vi "Update ROI times.vi"(11 "ROI setup in":T1[](array[typedef]) {"ROI group ID" format="%#_6f"; "Laser Power (%)" format="%#_6f"; "Zoom" format="%#_6f"; "Frame Size" format="%#_6f"; "Number of lines" format="%#_6f"; "Composite ID" format="%#_6f"; "Angle (deg)" format="%#_6f"; "ROI Time (ns)" format="%#_6f"; "ROI ID" format="%#_6f"; "Pixels in ROI" format="%#_6f"; "ROI index" format="%#_6f"; "Z stop" format="%#_6f"; "Y stop" format="%#_6f"; "X stop" format="%#_6f"; "Z start" format="%#_6f"; "X start" format="%#_6f"; "Y start" format="%#_6f"}) -> (3 "ROI setup out":T1[](array[typedef]) {"ROI group ID" format="%#_6f"; "Laser Power (%)" format="%#_6f"; "Zoom" format="%#_6f"; "Frame Size" format="%#_6f"; "Number of lines" format="%#_6f"; "Composite ID" format="%#_6f"; "Angle (deg)" format="%#_6f"; "ROI Time (ns)" format="%#_6f"; "ROI ID" format="%#_6f"; "Pixels in ROI" format="%#_6f"; "ROI index" format="%#_6f"; "Z stop" format="%#_6f"; "Y stop" format="%#_6f"; "X stop" format="%#_6f"; "Z start" format="%#_6f"; "X start" format="%#_6f"; "Y start" format="%#_6f"})   [LabVIEW 2013]
uses:
  Visualisation/Functional Imaging Viewer/Typedefs/ROI parameters data type.ctl
  Typedefs/ROI ID Enum.ctl
  ROI Entry screen/Globals/gl_ROI Entry UI globals.vi
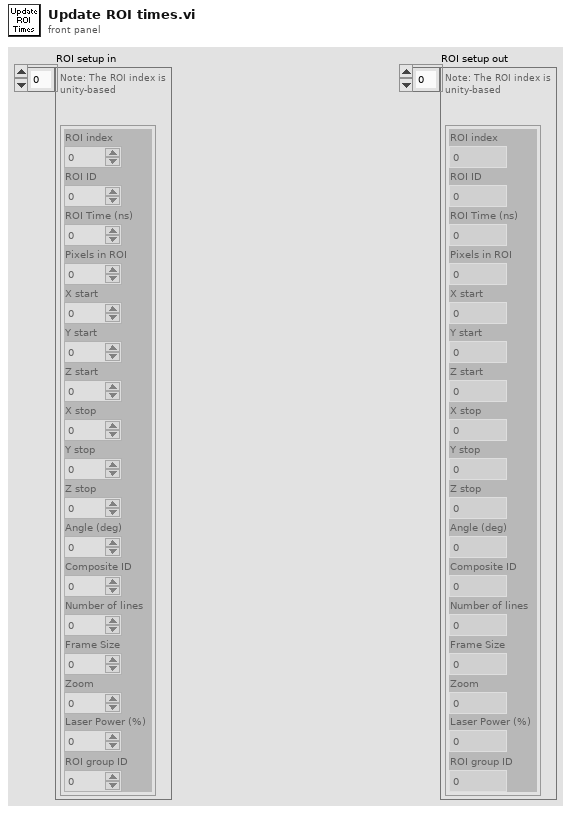
[diagram p1: front panel]
types:
  T1 = typedef "ROI parameters data type.ctl" = cluster{"ROI index":dbl, "ROI ID":dbl, "ROI Time (ns)":dbl, "Pixels in ROI":dbl, "X start":dbl, "Y start":dbl, "Z start":dbl, "X stop":dbl, "Y stop":dbl, "Z stop":dbl, "Angle (deg)":dbl, "Composite ID":dbl, "Number of lines":dbl, "Frame Size":dbl, "Zoom":dbl, "Laser Power (%)":dbl, "ROI group ID":dbl}
  T2 = typedef "ROI entry screen ctrl refs cluster.ctl" = cluster{"Done button":refnum<vi>, "Imaging button":refnum<vi>, "Acquisition button":refnum<vi>, "POI dwell time (us)":refnum<vi>, "Scan dwell time per pixel (us)":refnum<vi>, "# of planes":refnum<vi>, "Zoom":refnum<vi>, "Equal size":refnum<vi>, "Channel":refnum<vi>, "Image Display":refnum<vi>, "Z-Plane Selector":refnum<vi>, "Number of lines left":refnum<vi>, "Z-stack folder path":refnum<vi>, "POI Density":refnum<vi>, "Arb Plane Entry":refnum<vi>, "Whole plane":refnum<vi>, "Clear Last":refnum<vi>, "Clear All":refnum<vi>, "Trial Length (sec)":refnum<vi>, "Palette Type":refnum<vi>, "Intensity slider":refnum<vi>, "# POI":refnum<vi>, "Max Z Proj":refnum<vi>, "Zplane ind":refnum<vi>, "Wavelength (nm)":refnum<vi>, "Number of Trials":refnum<vi>, "Funct stim.trig.enable":refnum<vi>, "Funct stim.trig.delay (s)":refnum<vi>, "Line Mode":refnum<vi>, "Step size (µm)":refnum<vi>, "ROI move mode":refnum<vi>, "Cool-down time (s)":refnum<vi>, "Enable cool-down time":refnum<vi>, "Motor Z ind. (um)":refnum<vi>, "AOL Z ind. (um)":refnum<vi>}
  T3 = typedef "ROI ID Enum.ctl" = enum16{"Point", "MiniScan", "Comp. MiniScan", "Rectangle", "Comp. volume", "Arb. plane point"}
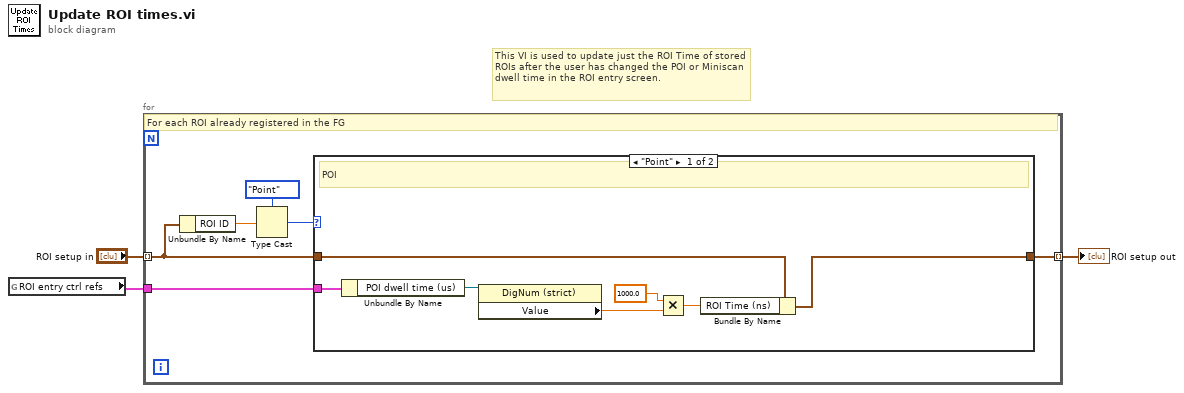
[diagram p0: block diagram]
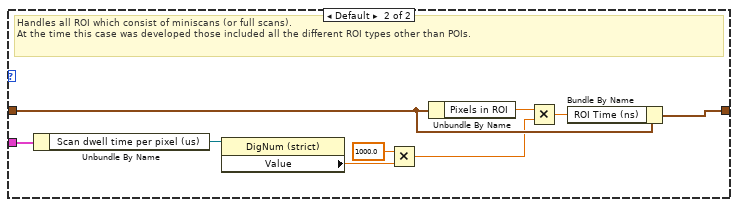
[diagram p2: hidden frame]
diagram:
  # "This VI is used to update just the ROI Time of stored ROIs after the user has changed the POI or Miniscan dwell time in the ROI entry screen."
  n1 = global read "gl_ROI Entry UI globals.vi" "ROI entry ctrl refs"() -> (w1:T2)
  n2 = for {
    tunnel: "ROI setup in" -> [w5] mode=indexing
    tunnel: [w9] -> w2 mode=indexing
    tunnel: w1 -> [w4]
    # "For each ROI already registered in the FG"
    n3 = Unbundle By Name(w5) -> ("ROI ID"=w7:dbl)
    n4 = Type Cast(type=ROI_ID_Enum."Point" ("ROI Type"), x=w7) -> (*(type *) &x=w6:T3)
    n5 = case shown="\"Point\"" w6 {
      tunnel: [w16 w24] -> w9
      tunnel: w5 -> [w15 w23]
      tunnel: w4 -> [w14 w21]
      frame "Point" {
        # "POI"
        n6 = Unbundle By Name(w14) -> ("POI dwell time (us)"=w13:refnum<vi>)
        n7 = property class="DigNum (strict)"(reference=w13) -> ("Value"=w11:dbl)  [unwired: 1 in, 2 out]
        n8 = Multiply(x=1000.0, y=w11) -> (x*y=w10:dbl)
        n9 = Bundle By Name(cluster=w15, "ROI Time (ns)"=w10) -> (w16:T1)
      }
      frame Default {
        # "Handles all ROI which consist of miniscans (or full scans).\nAt the time this case was developed those included all the different ROI types other than POIs."
        n10 = Unbundle By Name(w21) -> ("Scan dwell time per pixel (us)"=w22:refnum<vi>)
        n11 = property class="DigNum (strict)"(reference=w22) -> ("Value"=w19:dbl)  [unwired: 1 in, 2 out]
        n12 = Multiply(x=1000.0, y=w19) -> (x*y=w17:dbl)
        n13 = Unbundle By Name(w23) -> ("Pixels in ROI"=w18:dbl)
        n14 = Multiply(x=w18, y=w17) -> (x*y=w25:dbl)
        n15 = Bundle By Name(cluster=w23, "ROI Time (ns)"=w25) -> (w24:T1)
      }
    }
  }
  "ROI setup out" <- w2
